vi "Import Parameters Configuration File.vi"(8 "error in":errorcluster, 10 "parameters configuration file path":path caption="path to parameters xml", 11 "Ballard ARINC 429 custom device in":T1 format="%.0x") -> (0 "error out":errorcluster, 3 "Ballard ARINC 429 custom device out":T1 format="%.0x")   [LabVIEW 2020, in "Ballard ARINC 429 Scripting.lvlib"]
doc: "For the specified Ballard ARINC 429 custom device, imports the parameters configuration file located at the input <b>parameters configuration file path</b>. For successful deployment and operation, the parameters configuration must be consistent with the hardware configuration."
uses:
  Ballard ARINC 429 Scripting.lvlib
  <vilib>/NI VeriStand/Custom Device API/Custom Device Item Ref.ctl
  Import/ARINC 429 Import.lvlib
  <vilib>/NI VeriStand/Custom Device API/Custom Device API.lvlib
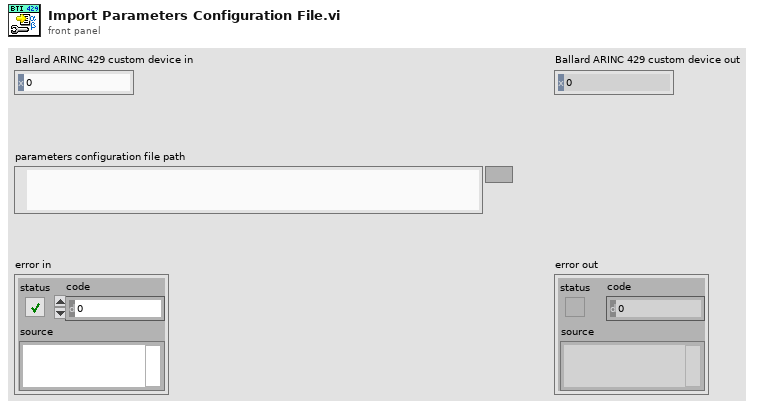
[diagram p1: front panel]
types:
  T1 = typedef "Custom Device API.lvlib/Custom Device Item Ref.ctl" = u64
  T2 = typedef "VS Channels Definition for All Labels on Hardware Channel.ctl" = cluster{"hardware channel":i32, "labels":T3[]}
  T3 = typedef "VS Channels Definition for Label.ctl" = cluster{"label (Dec)":u32, "parameters":T4[], "SDI value":u8, "SDI enabled":bool, "transfer type":T8, "create timestamp":bool}
  T4 = typedef "VS Channel Definition for Parameter.ctl" = cluster{"name":string, "direction":T5, "default value":dbl, "unit":string, "Parameter":T6}
  T5 = typedef "Direction.ctl" = enum16{"Rx", "Tx"}
  T6 = typedef "Parameter Definition.ctl" = cluster{"start index":i32, "size":i32, "encoding":T7, "signed":bool, "scale multiplier":dbl, "scale offset":dbl}
  T7 = typedef "Encoding and Decoding.lvlib/Encoding.ctl" = enum16{"BNR", "BCD", "Discrete"}
  T8 = typedef "Transfer Type.ctl" = enum16{"Scheduled", "Acyclic", "Block", "Strobe"}
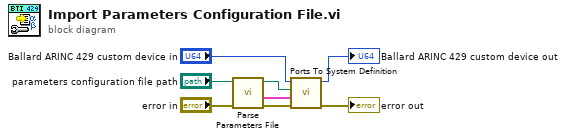
[diagram p0: block diagram]
diagram:
  n1 = call "Parse Parameters File.vi"("error in"="error in", "path to XML document"="parameters configuration file path") -> ("error out"=w8:errorcluster, "ports"=w7:T2[], "path to XML document out"=w6:path)  [unwired: 7 in]
  n2 = call "Ports To System Definition.vi"("error in"=w8, "ports"=w7, "parameter configuration file path"=w6, "custom device ref"="Ballard ARINC 429 custom device in") -> ("error out"=→"error out":errorcluster, "custom device ref out"=→"Ballard ARINC 429 custom device out":T1)  [unwired: 6 in]
